vi "Move.vi"(8 "error in (no error)":errorcluster, 10 "Up?":bool, 11 "PongPanel in":refnum<class "PongPanel.lvclass">) -> (0 "error out":errorcluster, 3 "PongPanel out":refnum<class "PongPanel.lvclass">)   [LabVIEW 2019, in "RT_Game.lvlib" / "PongPanel.lvclass"]
uses:
  PongPanel.lvclass
  C:/Users/FreshBob/Dropbox/VIs/myRIO_GameConsole/RT/RT_Game/GameObject/GameObject.lvclass
  GameObject/GameObject.lvclass/GameObject.ctl
  PongPanel.lvclass/PongPanel.ctl
  GameObject/Read position.vi
  GameObject/Read size.vi
  GameObject/Write position.vi
  Globals.vi
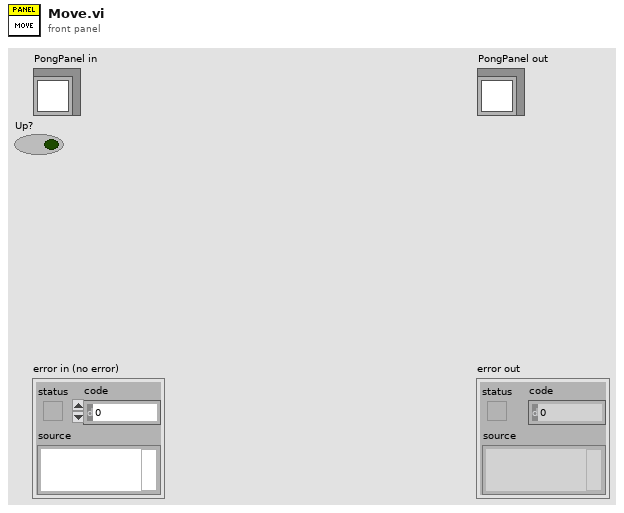
[diagram p1: front panel]
types:
  T1 = typedef "RT_Game.lvlib/Game.lvclass/Coordinate.ctl" = cluster{"x":dbl, "y":dbl}
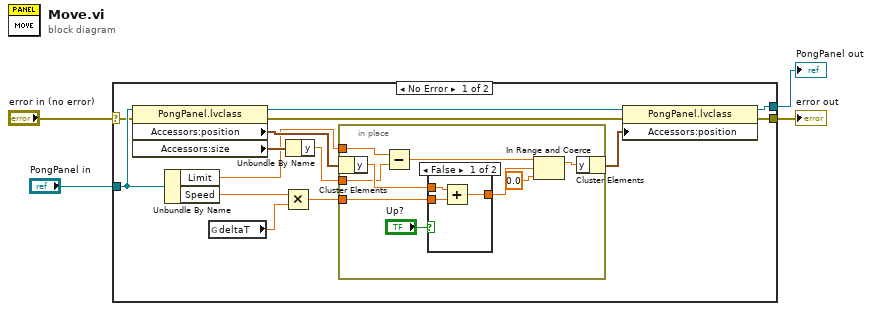
[diagram p0: block diagram]
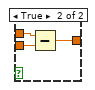
[diagram p2: hidden frame]
diagram:
  n1 = case shown="No Error" "error in (no error)" {
    selector: "error in (no error)" -> [w12 w35]
    tunnel: [w11 w35] -> w3
    tunnel: [w14 w34] -> w1
    tunnel: "PongPanel in" -> [w18 w34]
    frame No Error {
      n2 = property class="PongPanel.lvclass"(reference=w18, error in=w12) -> (reference out=w15:refnum<class "PongPanel.lvclass">, error out=w13:errorcluster, "Accessors:position"=w10:T1, "Accessors:size"=w7:T1)
      n3 = Unbundle By Name(w18) -> ("Limit"=w6:dbl, "Speed"=w17:dbl)
      n4 = global read "Globals.vi" "deltaT"() -> (w16:dbl)
      n5 = Multiply(x=w17, y=w16) -> (x*y=w8:dbl)
      n6 = Unbundle By Name(w7) -> ("y"=w5:dbl)
      n7 = in-place {
        in-place-border: w8 -> [w26]
        in-place-border: w6 -> [w21]
        in-place-border: w5 -> [w20]
        n8 = in-place-cluster #1(w10) -> ("y"=w27:dbl)
        n9 = Subtract(x=w21, y=w20) -> (x-y=w19:dbl)
        n10 = case shown="False" "Up?" {
          tunnel: w27 -> [w30 w33]
          tunnel: w26 -> [w29 w32]
          tunnel: [w28 w31] -> w25
          frame False {
            n11 = Add(x=w30, y=w29) -> (x+y=w28:dbl)
          }
          frame True {
            n12 = Subtract(x=w33, y=w32) -> (x-y=w31:dbl)
          }
        }
        n13 = In Range and Coerce(upper limit=w19, x=w25, lower limit=0.0) -> (coerced(x)=w23:dbl)  [unwired: 1 out]
        n14 = in-place-cluster #1("y"=w23) -> (w9:T1)
      }
      n15 = property class="PongPanel.lvclass"(reference=w15, error in=w13, "Accessors:position"=w9) -> (reference out=w14:refnum<class "PongPanel.lvclass">, error out=w11:errorcluster)
    }
    frame Error {
    }
  }
  "error out" <- w3
  "PongPanel out" <- w1
